vi "TON (Timer).vi"(7 "Reset":bool, 10 "Error In":errorcluster, 11 "Set Time":u32) -> (2 "Error Out":errorcluster, 3 "Timeout":bool, 5 "Elapsed Time":u32)   [LabVIEW 2019]
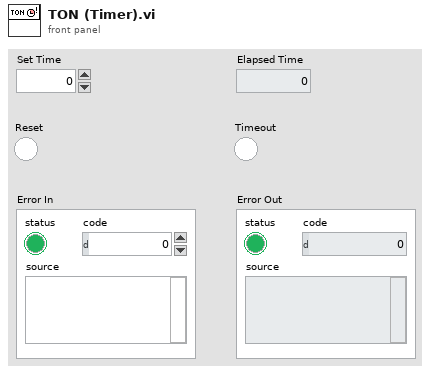
[diagram p1: front panel]
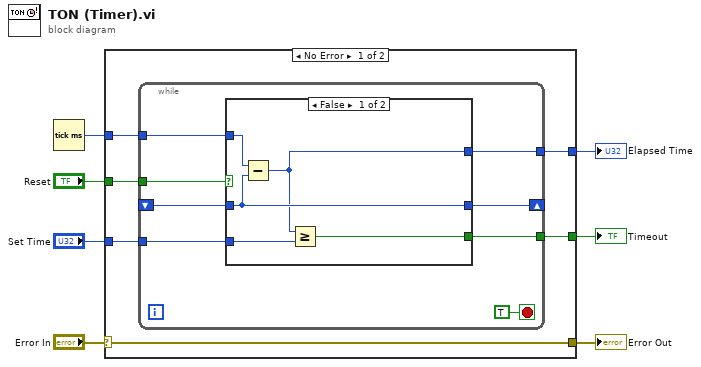
[diagram p0: block diagram]
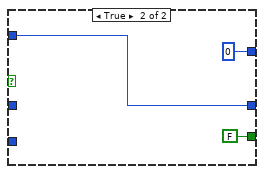
[diagram p2: hidden frame]
diagram:
  n1 = Tick Count (ms)() -> (millisecond timer value=w7:u32)
  n2 = case shown="No Error" "Error In" {
    selector: "Error In" -> [w8 w30]
    tunnel: w7 -> [w13 _]
    tunnel: "Reset" -> [w12 _]
    tunnel: [w11 _] -> w5
    tunnel: [w10 _] -> w4
    tunnel: "Set Time" -> [w9 _]
    tunnel: [w8 w30] -> w1
    frame No Error {
      n3 = while {
        tunnel: w13 -> [w21]
        shift-right: [w20] -> _
        shift-left: _ -> [w16]
        tunnel: w12 -> [w19]
        tunnel: [w18] -> w11
        tunnel: [w17] -> w10
        tunnel: w9 -> [w15]
        stop <- TRUE stop-if-true
        n4 = case shown="False" w19 {
          tunnel: w21 -> [w26 w29]
          tunnel: [w23 w29] -> w20
          tunnel: [w24 FALSE] -> w18
          tunnel: [w22 u32 0] -> w17
          tunnel: w16 -> [w23 _]
          tunnel: w15 -> [w25 _]
          frame False {
            n5 = Subtract(x=w26, y=w23) -> (x-y=w22:u32)
            n6 = Greater Or Equal?(x=w22, y=w25) -> (x >= y?=w24:bool)
          }
          frame True {
          }
        }
      }
    }
    frame Error {
    }
  }
  "Error Out" <- w1
  "Elapsed Time" <- w4
  "Timeout" <- w5
